vi "Acquire calibration sequence (SubVI).vi"(0 "Refnum in":T2, 1 "output cluster in":T4, 2 "Calibration \nruns":i32, 3 "Calibration framerate":i32, 5 "Measurement camera cluster in":T3, 7 "Measure \nintensities":bool, 9 "Transpose Measurement":bool, 11 "N samples":i32, 12 "ROI \nsize":dbl, 13 "Array":T2[](array[typedef]), 14 "Coordinate mapping \n(Monitor to Measurement)":T5) -> (4 "Numeric":i32)   [LabVIEW 2012]
uses:
  <vilib>/vision/Image Controls.llb/IMAQ Image.ctl
  Trap cluster.ctl
  <vilib>/userdefined/High Color/IMAQdx.ctl
  Get measurement coordinates.vi
  <vilib>/Utility/file.llb/Write To Spreadsheet File (DBL).vi
  <vilib>/vision/NI_Vision_Development_Module.lvlib
panel:
  in  "stop":bool
  out "Previous framerate":u32
  out "Waveform Graph":dbl[][](graph)
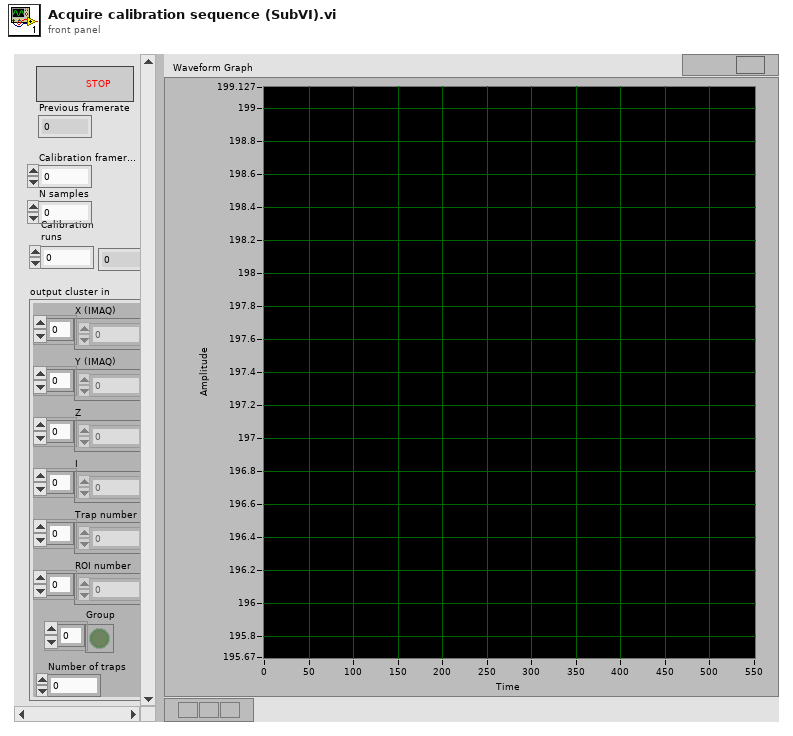
[diagram p1: front panel]
types:
  T1 = typedef "IMAQdx.ctl" = refnum<k21>
  T2 = typedef "IMAQ Image.ctl" = refnum<image>
  T3 = cluster{"Camera type":enum16{"IMAQ (Camera Link)", "IMAQ ring", "IMAQdx (firewire)", "No camera"}, "IMAQ Session":refnum<k11>, "IMAQdx Session":T1, "Image":T2, "Image buffers":T2[], "Camera error":errorcluster}
  T4 = typedef "Trap cluster.ctl" = cluster{"X (IMAQ)":sgl[], "Y (IMAQ)":sgl[], "Z":sgl[], "I":sgl[], "Trap number":i32[], "ROI number":i32[], "Number of traps":i32, "Group":bool[]}
  T5 = cluster{"cZ":sgl, "cY":sgl, "cX":sgl, "sZ":sgl, "sY":sgl, "sX":sgl}
  T6 = cluster{"CentroidX":dbl[], "CentroidY":dbl[], "I":dbl[], "Acquired Buffer Number":u32}
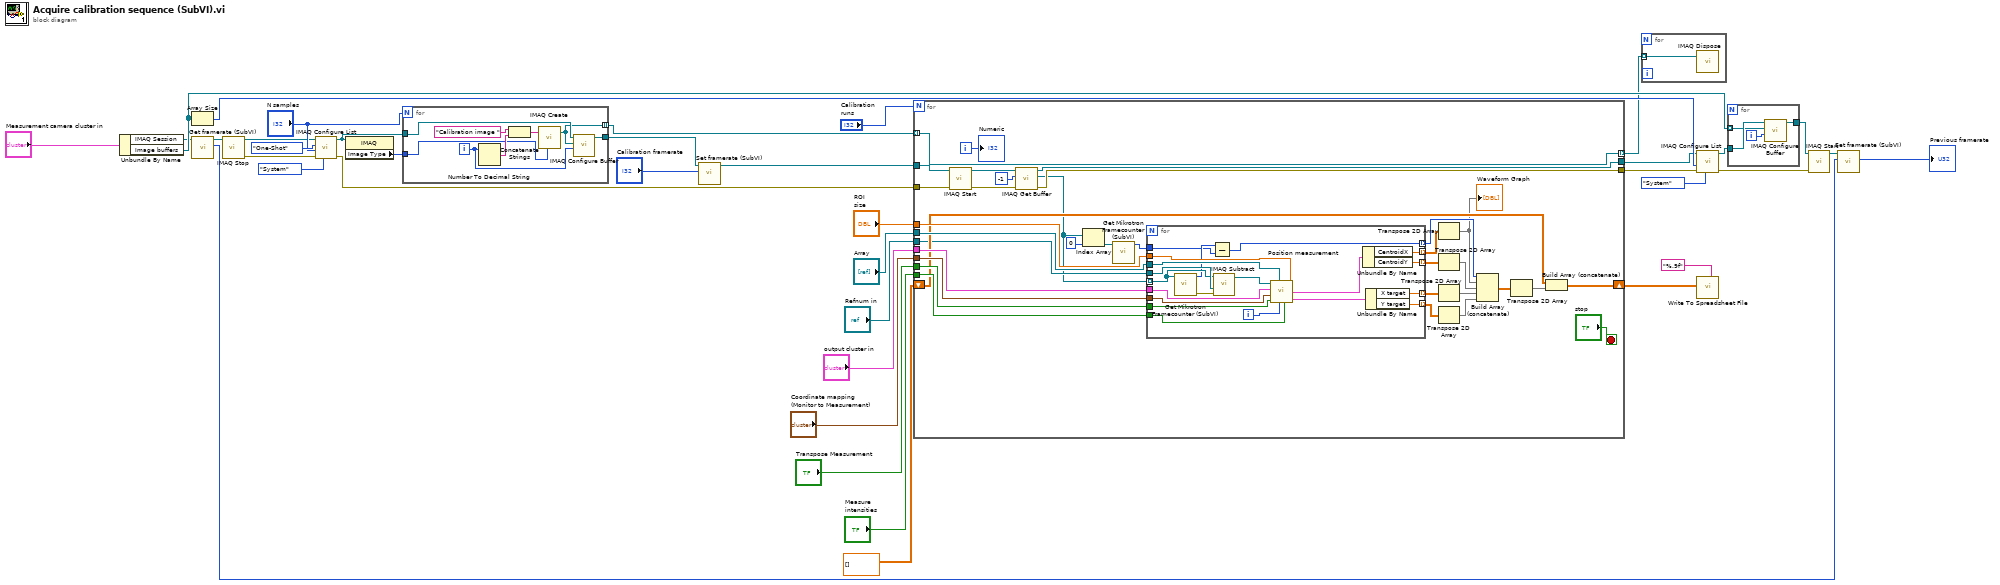
[diagram p0: block diagram]
diagram:
  n1 = Unbundle By Name("Measurement camera cluster in") -> ("IMAQ Session"=w3:refnum<k11>, "Image buffers"=w17:T2[])
  n2 = Array Size(array=w17) -> (size(s)=w16:i32)
  n3 = call "Get framerate (SubVI).vi"("IMAQ Refnum in"=w3) -> ("Current framerate"=w9:u32, "IMAQ Session Out"=w2:refnum<k11>)  [unwired: 8 in, 1 out]
  n4 = call <vilib>:"IMAQ Stop.vi"("IMAQ Session In"=w2) -> ("error out"=w20:errorcluster, "IMAQ Session Out"=w8:refnum<k11>)  [unwired: 9 in]
  n5 = call <vilib>:"IMAQ Configure List.vi"("Memory Location"=enum16{"System", "Onboard"}."System", "error in (no error)"=w20, "Number of buffers"="N samples", "Continuous?"=enum16{"One-Shot", "Continuous"}."One-Shot", "IMAQ Session In"=w8) -> ("error out"=w23:errorcluster, "IMAQ Session Out"=w14:refnum<k11>)  [unwired: 5 in]
  n6 = property class="IMAQ"(reference=w14) -> ("Image Type"=w13:u32)  [unwired: 1 in, 2 out]
  n7 = for {
    N: "N samples" -> [_]
    tunnel: w14 -> [w46]
    tunnel: w13 -> [w41]
    tunnel: [w40] -> w11 mode=indexing
    tunnel: [w39] -> w4
    i -> [w42]
    n8 = Number To Decimal String(number=w42) -> (decimal integer string=w44:string)  [unwired: 1 in]
    n9 = Concatenate Strings("Calibration image ", w44) -> (w43:string)
    n10 = call "IMAQ Create"("Image Name"=w43, "Image Type"=w41) -> ("New Image"=w40:T2)  [unwired: 3 in, 1 out]
    n11 = call <vilib>:"IMAQ Configure Buffer.vi"("Buffer Number"=w42, "Image In"=w40, "IMAQ Session In"=w46) -> ("IMAQ Session Out"=w39:refnum<k11>)  [unwired: 7 in, 1 out]
  }
  n12 = call "Set framerate (SubVI).vi"("Framerate"="Calibration framerate", "IMAQ Refnum in"=w4) -> ("IMAQ Session Out"=w7:refnum<k11>)  [unwired: 7 in, 2 out]
  n13 = for {
    N: "Calibration \nruns" -> [_]
    tunnel: w7 -> [w80]
    tunnel: w23 -> [w79]
    tunnel: [w75] -> w6
    tunnel: [w74] -> w24
    tunnel: "Array" -> [w73]
    tunnel: "output cluster in" -> [w72]
    tunnel: "Coordinate mapping \n(Monitor to Measurement)" -> [w71]
    tunnel: "Transpose Measurement" -> [w70]
    tunnel: "ROI \nsize" -> [w69]
    tunnel: "Measure \nintensities" -> [w68]
    shift-right: [w54] -> w35
    shift-left: dbl[][] [] -> [w58]
    tunnel: "Refnum in" -> [w55]
    tunnel: [w52] -> w12 mode=indexing
    tunnel: w11 -> [w52] mode=indexing
    i -> [w56]
    stop <- "stop" stop-if-true
    n14 = call <vilib>:"IMAQ Start.vi"("error in (no error)"=w79, "IMAQ Session In"=w80) -> ("error out"=w77:errorcluster, "IMAQ Session Out"=w78:refnum<k11>)  [unwired: 8 in]
    n15 = call <vilib>:"IMAQ Get Buffer.vi"("error in (no error)"=w77, "Buffer Number (-1:all)"=-1, "IMAQ Session In"=w78) -> ("error out"=w74:errorcluster, "Images Out"=w50:T2[], "IMAQ Session Out"=w75:refnum<k11>)  [unwired: 4 in, 2 out]
    n16 = Index Array(array=w50, index=0) -> (element=w49:T2)
    n17 = call "Get Mikrotron Framecounter (SubVI).vi"("Refnum in"=w49) -> ("Numeric"=w47:u32)  [unwired: 9 in, 1 out]
    n18 = for {
      tunnel: w73 -> [w100]
      tunnel: w50 -> [w85] mode=indexing
      tunnel: w72 -> [w99]
      tunnel: w71 -> [w98]
      tunnel: w70 -> [w97]
      tunnel: w69 -> [w86]
      tunnel: w68 -> [w96]
      tunnel: [w83] -> w63 mode=indexing
      tunnel: [w93] -> w62 mode=indexing
      tunnel: [w92] -> w61 mode=indexing
      tunnel: [w90] -> w60 mode=indexing
      tunnel: [w89] -> w59 mode=indexing
      tunnel: w55 -> [w88]
      tunnel: w47 -> [w81]
      i -> [w94]
      n19 = call "Get Mikrotron Framecounter (SubVI).vi"("Refnum in"=w85) -> ("error out"=w84:errorcluster, "Numeric"=w82:u32)  [unwired: 9 in]
      n20 = Subtract(x=w82, y=w81) -> (x-y=w83:u32)
      n21 = call "IMAQ Subtract"("Image Src A"=w85, "Image Src B"=w88, "error in (no error)"=w84) -> ("Image Dst Out"=w87:T2)  [unwired: 4 in, 1 out]
      n22 = call "Position measurement.vi"("Measure \nintensities"=w96, "ROI size"=w86, "Acquired Buffer Number"=w94, "Switch xy"=w97, "Coordinate mapping \n(Monitor to Measurement)"=w98, "ROIs"=w100, "Target positions (monitor)"=w99, "Image"=w87) -> ("Target coordinates (measurement)"=w91:cluster{"X target":sgl[], "Y target":sgl[]}, "Position data out (measurement)"=w95:T6)  [unwired: 1 in]
      n23 = Unbundle By Name(w95) -> ("CentroidX"=w93:dbl[], "CentroidY"=w92:dbl[])
      n24 = Unbundle By Name(w91) -> ("X target"=w90:sgl[], "Y target"=w89:sgl[])
    }
    n25 = Transpose 2D Array(2D array=w62) -> (transposed array=w53:dbl[][])
    "Waveform Graph" <- w53
    n26 = Transpose 2D Array(2D array=w61) -> (transposed array=w67:dbl[][])
    n27 = Transpose 2D Array(2D array=w60) -> (transposed array=w66:sgl[][])
    n28 = Transpose 2D Array(2D array=w59) -> (transposed array=w65:sgl[][])
    n29 = Build Array (concatenate)(w63, w53, w67, w66, w65) -> (w64:dbl[][])
    n30 = Transpose 2D Array(2D array=w64) -> (transposed array=w57:dbl[][])
    n31 = Build Array (concatenate)(w58, w57) -> (w54:dbl[][])
    "Numeric" <- w56
  }
  n32 = for {
    tunnel: w12 -> [w101] mode=indexing
    n33 = call "IMAQ Dispose"("Image"=w101) -> ()  [unwired: 5 in, 1 out]
  }
  n34 = call <vilib>:"IMAQ Configure List.vi"("Memory Location"=enum16{"System", "Onboard"}."System", "error in (no error)"=w24, "Number of buffers"=w16, "IMAQ Session In"=w6) -> ("error out"=w25:errorcluster, "IMAQ Session Out"=w19:refnum<k11>)  [unwired: 6 in]
  n35 = call-poly <vilib>:"Write To Spreadsheet File.vi"("format (%.3f)"="%.9f", "2D data"=w35) -> ()  [unwired: 6 in, 1 out]
  n36 = for {
    tunnel: w19 -> [w105]
    tunnel: [w104] -> w18
    tunnel: w17 -> [w103] mode=indexing
    i -> [w102]
    n37 = call <vilib>:"IMAQ Configure Buffer.vi"("Buffer Number"=w102, "Image In"=w103, "IMAQ Session In"=w105) -> ("IMAQ Session Out"=w104:refnum<k11>)  [unwired: 7 in, 1 out]
  }
  n38 = call <vilib>:"IMAQ Start.vi"("error in (no error)"=w25, "IMAQ Session In"=w18) -> ("IMAQ Session Out"=w5:refnum<k11>)  [unwired: 8 in, 1 out]
  n39 = call "Set framerate (SubVI).vi"("Framerate"=w9, "IMAQ Refnum in"=w5) -> ("Current framerate"=→"Previous framerate":u32)  [unwired: 7 in, 2 out]
